vi "LaserCal-Update Sequence (I-O).vi"(0 "Runtime State":T1, 7 "SeqVal":dbl, 9 "Start?":bool=TRUE, 11 "error in (no error)":errorcluster) -> (15 "error out":errorcluster)   [LabVIEW 2015]
uses:
  Typedefs/LaserCal-Meter Runtime State.ctl
  Typedefs/LaserCal-Meter Stimulus.ctl
  Typedefs/LaserCal-Control Mode.ctl
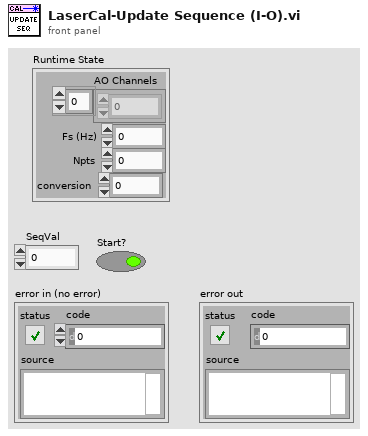
[diagram p1: front panel]
types:
  T1 = typedef "LaserCal-Meter Runtime State.ctl" = cluster{"AO Channels":i32[], "Fs (Hz)":dbl, "Npts":i32, "conversion":dbl}
  T2 = typedef "LaserCal-Meter Stimulus.ctl" = cluster{"Vcommand":dbl, "scale":enum16{"linear", "dB"}, "Pulsed":bool, "Pulse width (ms)":dbl, "Pulse rate (Hz)":dbl, "mode":T3}
  T3 = typedef "LaserCal-Control Mode.ctl" = enum16{"Voltage only", "Voltage + Enable"}
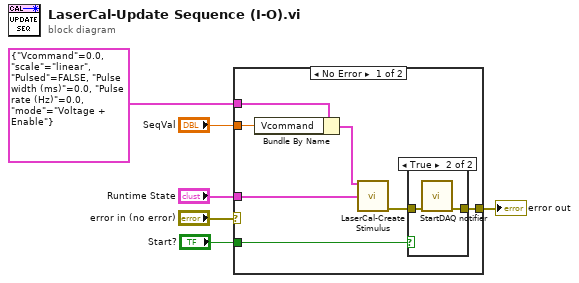
[diagram p0: block diagram]
diagram:
  n1 = case shown="No Error" "error in (no error)" {
    selector: "error in (no error)" -> [_ w17]
    tunnel: [w8 w17] -> w3
    tunnel: "SeqVal" -> [w10 _]
    tunnel: "Runtime State" -> [w12 _]
    tunnel: T2 {"Vcommand"=0.0, "scale"=enum."linear", "Pulsed"=FALSE, "Pulse width (ms)"=0.0, "Pulse rate (Hz)"=0.0, "mode"=enum."Voltage + Enable"} ("Stimulus (I-O)") -> [w11 _]
    tunnel: "Start?" -> [w7 _]
    frame No Error {
      n2 = Bundle By Name(cluster=w11, "Vcommand"=w10) -> (w9:T2)
      n3 = call "LaserCal-Create Stimulus.vi"("Stimulus"=w9, "Runtime State"=w12) -> ("error out"=w13:errorcluster)  [unwired: 11 in, 2 out]
      n4 = case shown="True" w7 {
        tunnel: w13 -> [w14 w16]
        tunnel: [w14 w15] -> w8
        frame False {
        }
        frame True {
          n5 = call "StartDAQ notifier.vi"("error in (no error)"=w16) -> ("error out"=w15:errorcluster)  [unwired: 6 in]
        }
      }
    }
    frame Error {
    }
  }
  "error out" <- w3
